vi "Counter - Read Pulse Width and Frequency (Continuous).vi"() -> ()   [LabVIEW 2017]
doc: "本范例演示连续执行周期、频率、脉冲宽度，脉冲宽度，或两边沿间隔等类型测量的方法。\n\n本范例采用隐式定时，即输入信号的每个周期采集一个采样。\n\n关于将信号连接至DAQ设备的方法，可参考设备文档。"
uses:
  <vilib>/Utility/error.llb/DialogType.ctl
  <vilib>/DAQmx/read.llb/DAQmx Read (Counter 1D DBL 1Chan NSamp).vi
  <vilib>/DAQmx/create/channels.llb/DAQmx Create Channel (CI-Period).vi
  <vilib>/DAQmx/create/channels.llb/DAQmx Create Channel (CI-Frequency).vi
  <vilib>/DAQmx/create/channels.llb/DAQmx Create Channel (CI-Pulse Width).vi
  <vilib>/DAQmx/create/channels.llb/DAQmx Create Channel (CI-Two Edge Separation).vi
  <vilib>/DAQmx/configure/timing.llb/DAQmx Timing (Implicit).vi
  <vilib>/DAQmx/miscellaneous.llb/DAQmx Fill In Error Info.vi
  <resource>/objmgr/daqmx.rc
panel:
  out "数据":dbl[](array[numeric])
  in  "计数器输入类型":T1(tab)
  in  "周期输入接线端":tag="/Dev1/PFI9"
  in  "最大周期":dbl=0.1 format="%0.6f"
  in  "最小周期":dbl=1e-06 format="%0.6f"
  in  "最小频率":dbl=2.0 format="%0.6f"
  in  "最大频率":dbl=100.0 format="%0.6f"
  in  "频率输入接线端":tag="/Dev1/PFI9"
  in  "脉冲宽度输入接线端":tag="/Dev1/PFI9"
  in  "最小脉冲宽度":dbl=1e-06 format="%0.6f"
  in  "最大脉冲宽度":dbl=0.1 format="%0.6f"
  in  "第二个输入信号":tag="/Dev1/PFI9"
  in  "第一个输入接线端":tag="/Dev1/PFI10"
  in  "最小间隔时间":dbl=1e-06 format="%0.6f"
  in  "最大间隔时间":dbl=0.1 format="%0.6f"
  in  "停止":bool
  in  "每次循环采样数":i32=1000
  in  "计数器":tag="Dev1/ctr0"
  # "通道设置"
  # "采集数据"
  # "定时设置"
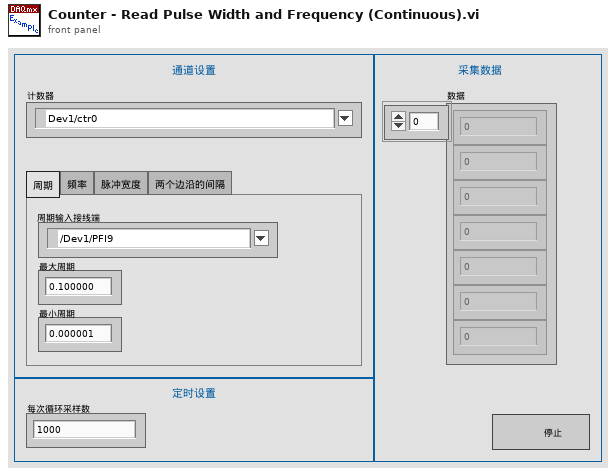
[diagram p1: front panel]
types:
  T1 = enum32{"Period", "Frequency", "Pulse Width", "2 Edge Separation"}
  T2 = typedef "DialogType.ctl" = u16
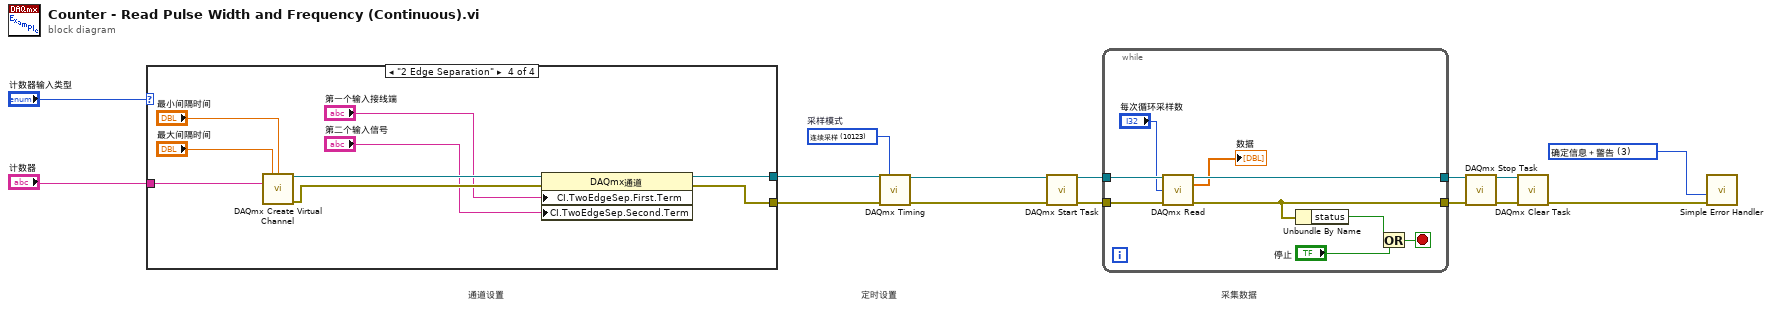
[diagram p0: block diagram]
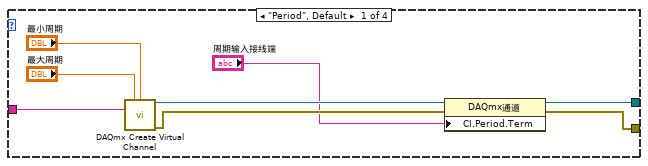
[diagram p2: hidden frame]
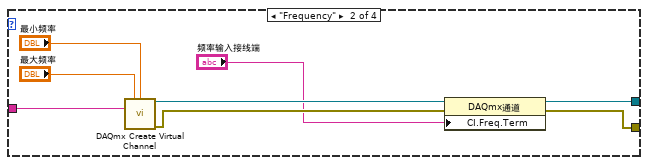
[diagram p3: hidden frame]
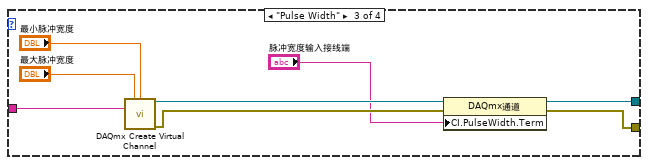
[diagram p4: hidden frame]
diagram:
  w1 = T2 3 items=["无对话框", "确定信息", "继续或停止信息", "确定信息＋警告", "继续/停止＋警告"] ("对话框类型（确定信息：1）")
  w15 = 10123 items=["有限采样"=10178, "连续采样"=10123, "硬件定时单点"=12522]  # 采样模式
  # "采集数据"
  # "定时设置"
  # "通道设置"
  n1 = case shown="\"2 Edge Separation\"" "计数器输入类型" {
    tunnel: [w21 w29 w37 w46] -> w14
    tunnel: [w22 w30 w38 w47] -> w13
    tunnel: "计数器" -> [w23 w31 w39 w48]
    frame "Period", Default {
      n2 = call-poly <vilib>:"DAQmx Create Virtual Channel.vi"("maximum value"="最大周期", "minimum value"="最小周期", "counter"=w23) -> ("task out"=w20:refnum<k21>, "error out"=w19:errorcluster)  [unwired: 11 in]
      n3 = property class="DAQmx通道"(reference=w20, error in=w19, "CI.Period.Term"="周期输入接线端") -> (reference out=w22:refnum<k21>, error out=w21:errorcluster)
    }
    frame "Frequency" {
      n4 = call-poly <vilib>:"DAQmx Create Virtual Channel.vi"("maximum value"="最大频率", "minimum value"="最小频率", "counter"=w31) -> ("task out"=w28:refnum<k21>, "error out"=w27:errorcluster)  [unwired: 11 in]
      n5 = property class="DAQmx通道"(reference=w28, error in=w27, "CI.Freq.Term"="频率输入接线端") -> (reference out=w30:refnum<k21>, error out=w29:errorcluster)
    }
    frame "Pulse Width" {
      n6 = call-poly <vilib>:"DAQmx Create Virtual Channel.vi"("maximum value"="最大脉冲宽度", "minimum value"="最小脉冲宽度", "counter"=w39) -> ("task out"=w36:refnum<k21>, "error out"=w35:errorcluster)  [unwired: 11 in]
      n7 = property class="DAQmx通道"(reference=w36, error in=w35, "CI.PulseWidth.Term"="脉冲宽度输入接线端") -> (reference out=w38:refnum<k21>, error out=w37:errorcluster)
    }
    frame "2 Edge Separation" {
      n8 = call-poly <vilib>:"DAQmx Create Virtual Channel.vi"("maximum value"="最大间隔时间", "minimum value"="最小间隔时间", "counter"=w48) -> ("task out"=w45:refnum<k21>, "error out"=w44:errorcluster)  [unwired: 11 in]
      n9 = property class="DAQmx通道"(reference=w45, error in=w44, "CI.TwoEdgeSep.First.Term"="第一个输入接线端", "CI.TwoEdgeSep.Second.Term"="第二个输入信号") -> (reference out=w47:refnum<k21>, error out=w46:errorcluster)
    }
  }
  n10 = call-poly <vilib>:"DAQmx Timing.vi"("task/channels in"=w13, "sample mode"=w15, "error in"=w14) -> ("task out"=w7:refnum<k21>, "error out"=w6:errorcluster)  [unwired: 11 in]
  n11 = call <vilib>:"DAQmx Start Task.vi"("task/channels in"=w7, "error in"=w6) -> ("task out"=w12:refnum<k21>, "error out"=w11:errorcluster)  [unwired: 12 in]
  n12 = while {
    tunnel: w12 -> [w57]
    tunnel: w11 -> [w56]
    tunnel: [w53] -> w2
    tunnel: [w54] -> w3
    stop <- w55 stop-if-true
    n13 = call-poly <vilib>:"DAQmx Read.vi"("task/channels in"=w57, "number of samples per channel"="每次循环采样数", "error in"=w56) -> ("task out"=w54:refnum<k21>, "data"=→"数据":dbl[], "error out"=w53:errorcluster)  [unwired: 10 in]
    n14 = Unbundle By Name(w53) -> ("status"=w52:bool)
    n15 = Or(x=w52, y="停止") -> (x .or. y?=w55:bool)
  }
  n16 = call <vilib>:"DAQmx Stop Task.vi"("task/channels in"=w3, "error in"=w2) -> ("task out"=w5:refnum<k21>, "error out"=w4:errorcluster)  [unwired: 12 in]
  n17 = call <vilib>:"DAQmx Clear Task.vi"("task in"=w5, "error in"=w4) -> ("error out"=w10:errorcluster)  [unwired: 13 in]
  n18 = call <vilib>:"Simple Error Handler.vi"("type of dialog (OK msg:1)"=w1, "error in (no error)"=w10) -> ()  [unwired: 3 in, 5 out]
